vi "Create Server from Template.vi"(8 "error in (no error)":errorcluster, 9 "Generated Server Name":string="Generated Server", 10 "Target Project Path":path, 11 "Application ref in":refnum<vi>) -> (0 "error out":errorcluster, 1 "Already exists ?":bool, 2 "Server class out":refnum<vi>, 3 "Server library out":refnum<vi>)   [LabVIEW 2019, in "gRPC Scripting Tools.lvlib"]
uses:
  gRPC Scripting Tools.lvlib
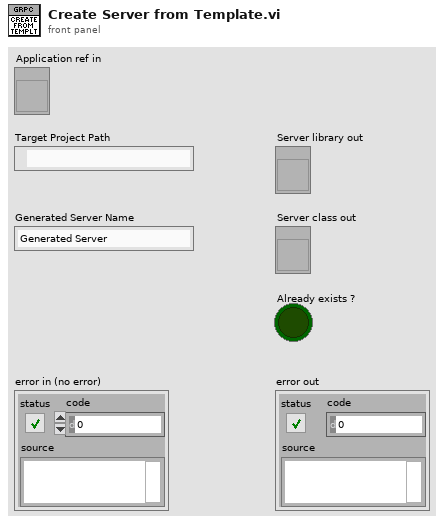
[diagram p1: front panel]
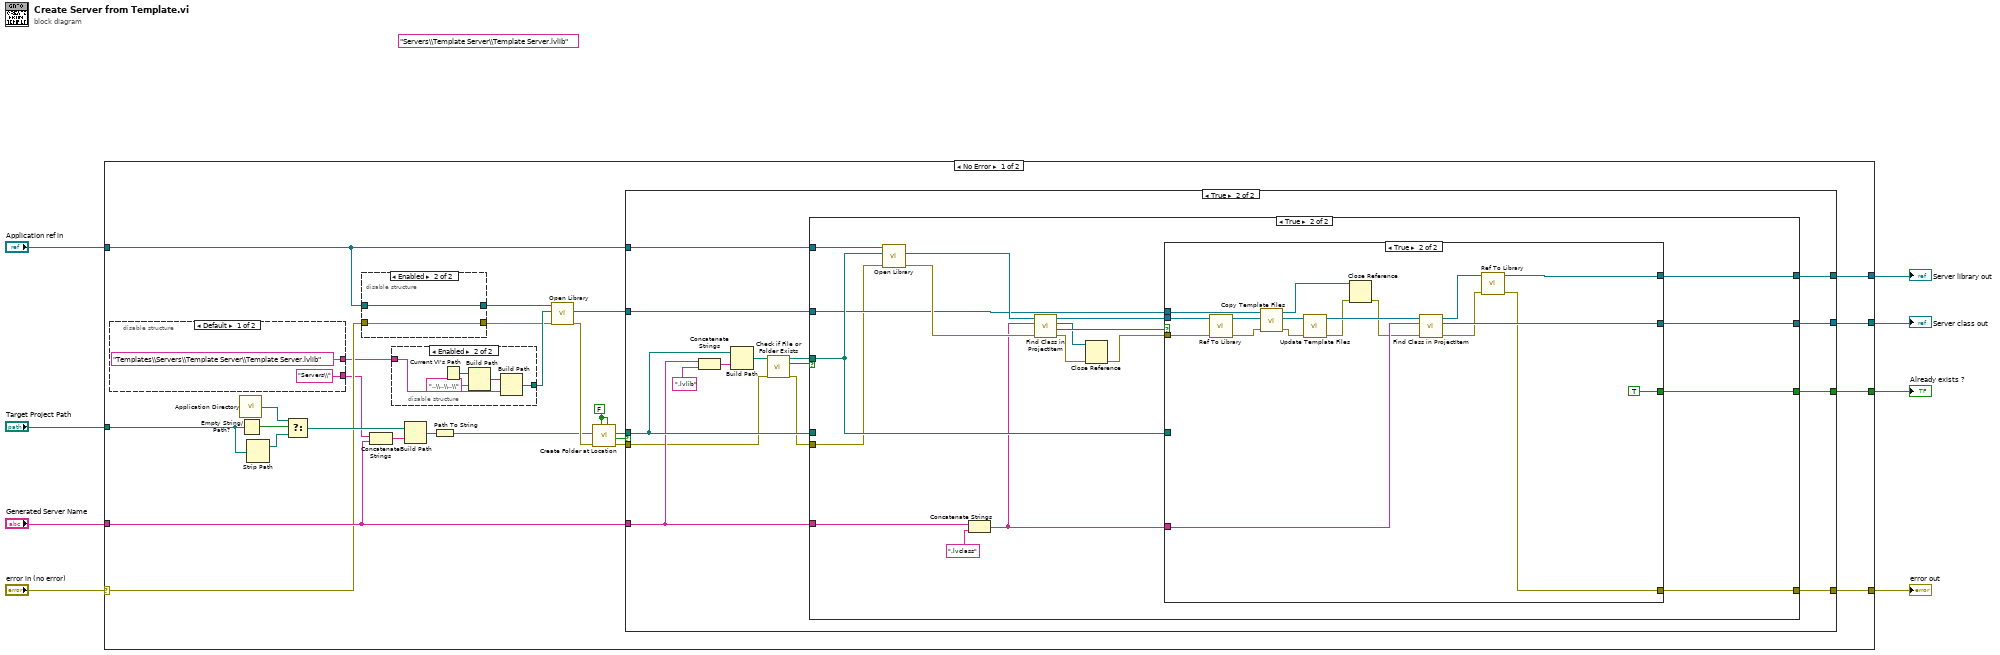
[diagram p0: block diagram]
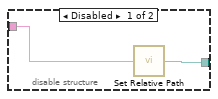
[diagram p2: hidden frame]
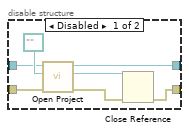
[diagram p3: hidden frame]
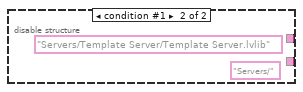
[diagram p4: hidden frame]
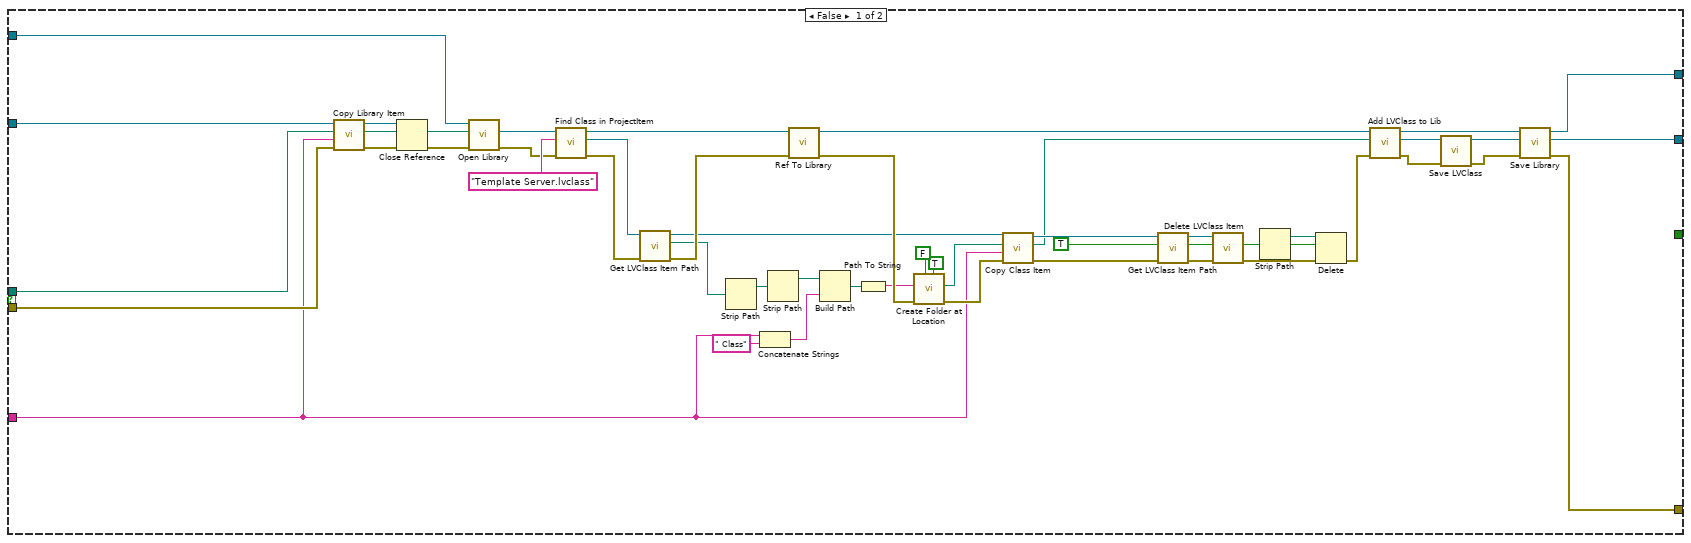
[diagram p5: hidden frame]
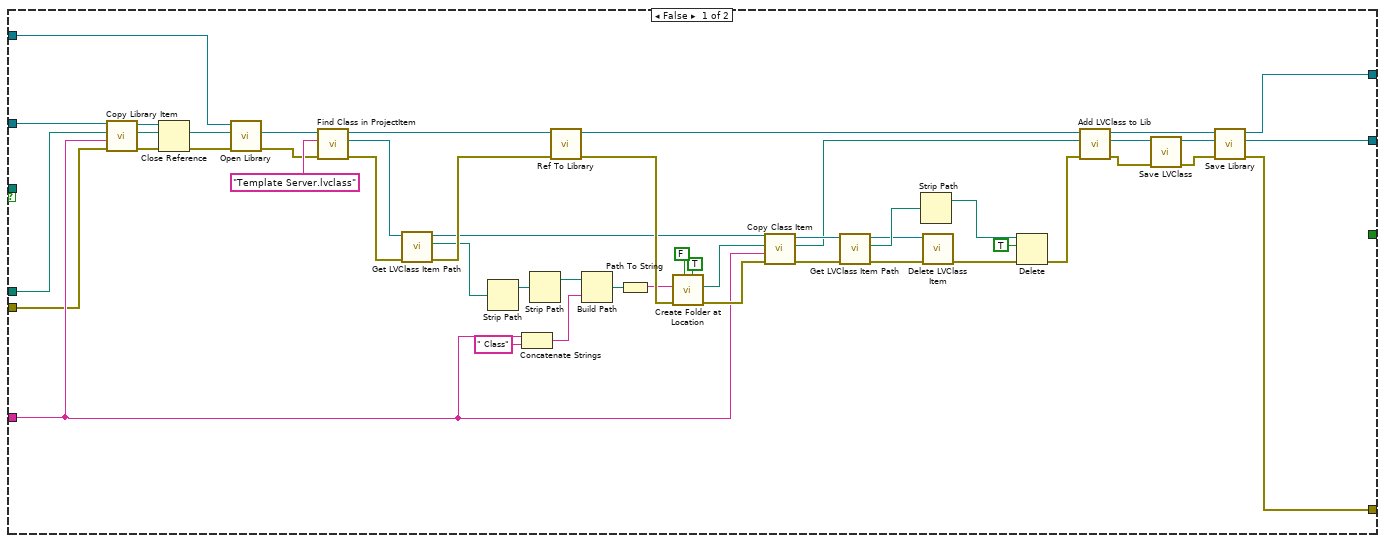
[diagram p6: hidden frame]
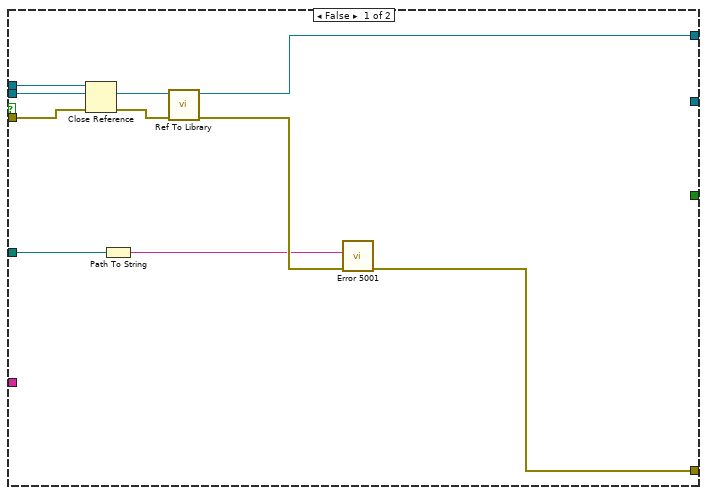
[diagram p7: hidden frame]
diagram:
  (unwired) "Servers\\Template Server\\Template Server.lvlib" ("Application Relative Path")
  n1 = case shown="No Error" "error in (no error)" {
    selector: "error in (no error)" -> [w13 w207]
    tunnel: [w34 w207] -> w8
    tunnel: [w33 _] -> w7
    tunnel: [w32 _] -> w6
    tunnel: "Target Project Path" -> [w16 _]
    tunnel: "Generated Server Name" -> [w15 _]
    tunnel: "Application ref in" -> [w14 _]
    tunnel: [w11 _] -> w1
    frame No Error {
      w25 = FALSE ("Use Relative")
      n2 = disable-structure shown="Default" {
        disable-tunnel: ["Templates\\Servers\\Template Server\\Template Server.lvlib" ("Application Relative Path") _] -> w10
        disable-tunnel: ["Servers\\" ("Path") _] -> w9
        frame condition #0 (active) {
        }
        frame condition #1 {
          (unwired) "Servers/" ("Path")
          (unwired) "Servers/Template Server/Template Server.lvlib" ("Application Relative Path")
        }
      }
      n3 = call <vilib>:"Application Directory.vi"() -> ("Application Directory"=w17:path)
      n4 = Empty String/Path?(string/path=w16) -> (empty?=w20:bool)
      n5 = Strip Path(path=w16) -> (stripped path=w19:path)  [unwired: 1 out]
      n6 = Select(t=w17, s=w20, f=w19) -> (s? t:f=w18:path)
      n7 = disable-structure shown="Enabled" {
        disable-tunnel: [w48 w50] -> w28
        disable-tunnel: [w45 w49] -> w21
        disable-tunnel: w14 -> [w43 w50]
        disable-tunnel: w13 -> [w42 w49]
        frame Disabled {
          n8 = call "Open Project.vi"("error in (no error)"=w42, "Project Path in"=path "", "Application reference"=w43) -> ("error out"=w46:errorcluster, "Project out"=w47:refnum<vi>, "Application out"=w48:refnum<vi>)  [unwired: 6 in]
          n9 = Close Reference(reference=w47, error in (no error)=w46) -> (error out=w45:errorcluster)
        }
        frame Enabled {
        }
      }
      n10 = Concatenate Strings(w9, w15) -> (w24:string)
      n11 = disable-structure shown="Enabled" {
        disable-tunnel: [w36 w39] -> w29
        disable-tunnel: w10 -> [w35 w37]
        frame Disabled {
          n12 = call "Set Relative Path.vi"("Application Relative Path"=w35) -> ("Full Path"=w36:path)
        }
        frame Enabled {
          n13 = Current VI's Path() -> (path=w41:path)
          n14 = Build Path(base path=w41, name or relative path="..\\..\\..\\") -> (appended path=w38:path)
          n15 = Build Path(base path=w38, name or relative path=w37) -> (appended path=w39:path)
        }
      }
      n16 = Build Path(base path=w18, name or relative path=w24) -> (appended path=w23:path)
      n17 = Path To String(path=w23) -> (string=w22:string)
      n18 = call "Open Library.vi"("error in (no error)"=w21, "Full Path"=w29, "Application in"=w28) -> ("error out"=w30:errorcluster, "Library out"=w26:refnum<vi>)  [unwired: 6 in, 1 out]
      n19 = call "Create Folder at Location.vi"("Override existing (F)"=w25, "Use Relative (F)"=w25, "Error In"=w30, "Path"=w22) -> ("Error Out"=w31:errorcluster, "Already Exists ?"=w12:bool, "Full path out"=w27:path)  [unwired: 5 in]
      n20 = case shown="True" w12 {
        tunnel: [w99 w104] -> w34
        tunnel: [w98 w109] -> w33
        tunnel: [w97 w110] -> w32
        tunnel: w31 -> [w61 w101]
        tunnel: w27 -> [w60 w106]
        tunnel: w26 -> [w59 w107]
        tunnel: w15 -> [w54 w105]
        tunnel: w14 -> [w53 w108]
        tunnel: [_ w103] -> w11
        frame False {
          n21 = call "Copy Library Item.vi"("error in (no error)"=w61, "Copy Name"=w54, "Copy location"=w60, "Library in"=w59) -> ("error out"=w82:errorcluster, "New Lib Path"=w58:path, "Library out"=w81:refnum<vi>)  [unwired: 5 in]
          n22 = Close Reference(reference=w81, error in (no error)=w82) -> (error out=w57:errorcluster)
          n23 = call "Open Library.vi"("error in (no error)"=w57, "Full Path"=w58, "Application in"=w53) -> ("error out"=w55:errorcluster, "Library out"=w56:refnum<vi>)  [unwired: 6 in, 1 out]
          n24 = call "Find Class in ProjectItem.vi"("error in (no error)"=w55, "Class Name"="Template Server.lvclass", "ProjectItem in"=w56) -> ("error out"=w64:errorcluster, "LVClass out"=w63:refnum<vi>, "ProjectItem out"=w76:refnum<vi>)  [unwired: 5 in, 1 out]
          n25 = call "Get LVClass Item Path.vi"("error in (no error)"=w64, "LVClassLibrary in"=w63) -> ("error out"=w78:errorcluster, "Path"=w65:path, "LVClassLibrary out"=w66:refnum<vi>)  [unwired: 7 in]
          n26 = Strip Path(path=w65) -> (stripped path=w74:path)  [unwired: 1 out]
          n27 = Concatenate Strings(w54, " Class" ("string")) -> (w69:string)
          n28 = Strip Path(path=w74) -> (stripped path=w75:path)  [unwired: 1 out]
          n29 = call "Ref To Library.vi"("error in (no error)"=w78, "ProjectItem in"=w76) -> ("error out"=w79:errorcluster, "Library out"=w92:refnum<vi>)  [unwired: 8 in]
          n30 = Build Path(base path=w75, name or relative path=w69) -> (appended path=w70:path)
          n31 = Path To String(path=w70) -> (string=w71:string)
          n32 = call "Create Folder at Location.vi"("Override existing (F)"=TRUE, "Use Relative (F)"=FALSE ("Use Relative"), "Error In"=w79, "Path"=w71) -> ("Error Out"=w80:errorcluster, "Full path out"=w73:path)  [unwired: 5 in, 1 out]
          n33 = call "Copy Class Item.vi"("error in (no error)"=w80, "New Name"=w54, "Full path in"=w73, "LVClassLibrary in"=w66) -> ("error out"=w84:errorcluster, "New Class Path out"=w77:path, "LVClassLibrary out"=w83:refnum<vi>)  [unwired: 5 in]
          n34 = call "Get LVClass Item Path.vi"("error in (no error)"=w84, "LVClassLibrary in"=w83) -> ("error out"=w86:errorcluster, "Path"=w87:path, "LVClassLibrary out"=w85:refnum<vi>)  [unwired: 7 in]
          n35 = call "Delete LVClass Item.vi"("error in (no error)"=w86, "LVClassLibrary in"=w85) -> ("error out"=w89:errorcluster)  [unwired: 9 in]
          n36 = Strip Path(path=w87) -> (stripped path=w88:path)  [unwired: 1 out]
          n37 = Delete(path (use dialog)=w88, entire hierarchy (F)=TRUE, error in=w89) -> (error out=w90:errorcluster)  [unwired: 2 in, 2 out]
          n38 = call "Add LVClass to Lib.vi"("error in (no error)"=w90, "LVClass Path in"=w77, "Library in"=w92) -> ("error out"=w95:errorcluster, "LVClassLibrary out"=w94:refnum<vi>, "Library out"=w93:refnum<vi>)  [unwired: 6 in]
          n39 = call "Save LVClass.vi"("error in (no error)"=w95, "LVClassLibrary in"=w94) -> ("error out"=w96:errorcluster, "LVClassLibrary out"=w98:refnum<vi>)  [unwired: 8 in]
          n40 = call "Save Library.vi"("error in (no error)"=w96, "Library in"=w93) -> ("error out"=w99:errorcluster, "Library out"=w97:refnum<vi>)  [unwired: 8 in]
        }
        frame True {
          n41 = Concatenate Strings(w105, ".lvlib" ("string")) -> (w113:string)
          n42 = Build Path(base path=w106, name or relative path=w113) -> (appended path=w112:path)
          n43 = call <vilib>:"Check if File or Folder Exists.vi"("error in (no error)"=w101, "path"=w112) -> ("error out"=w100:errorcluster, "file or folder exists?"=w111:bool, "dup path"=w102:path)  [unwired: 7 in]
          n44 = case shown="True" w111 {
            tunnel: [w122 w173] -> w110
            tunnel: [w121 w162] -> w109
            tunnel: w108 -> [w120 w179]
            tunnel: w107 -> [w119 w168]
            tunnel: w106 -> [w118 _]
            tunnel: w105 -> [w117 w177]
            tunnel: w100 -> [w116 w167]
            tunnel: [w115 w172] -> w104
            tunnel: [_ w170] -> w103
            tunnel: w102 -> [_ w169]
            frame False {
              n45 = call "Copy Library Item.vi"("error in (no error)"=w116, "Copy Name"=w117, "Copy location"=w118, "Library in"=w119) -> ("error out"=w147:errorcluster, "New Lib Path"=w126:path, "Library out"=w146:refnum<vi>)  [unwired: 5 in]
              n46 = Close Reference(reference=w146, error in (no error)=w147) -> (error out=w125:errorcluster)
              n47 = call "Open Library.vi"("error in (no error)"=w125, "Full Path"=w126, "Application in"=w120) -> ("error out"=w123:errorcluster, "Library out"=w124:refnum<vi>)  [unwired: 6 in, 1 out]
              n48 = call "Find Class in ProjectItem.vi"("error in (no error)"=w123, "Class Name"="Template Server.lvclass", "ProjectItem in"=w124) -> ("error out"=w129:errorcluster, "LVClass out"=w128:refnum<vi>, "ProjectItem out"=w141:refnum<vi>)  [unwired: 5 in, 1 out]
              n49 = call "Get LVClass Item Path.vi"("error in (no error)"=w129, "LVClassLibrary in"=w128) -> ("error out"=w143:errorcluster, "Path"=w130:path, "LVClassLibrary out"=w131:refnum<vi>)  [unwired: 7 in]
              n50 = Strip Path(path=w130) -> (stripped path=w139:path)  [unwired: 1 out]
              n51 = Concatenate Strings(w117, " Class" ("string")) -> (w134:string)
              n52 = Strip Path(path=w139) -> (stripped path=w140:path)  [unwired: 1 out]
              n53 = call "Ref To Library.vi"("error in (no error)"=w143, "ProjectItem in"=w141) -> ("error out"=w144:errorcluster, "Library out"=w157:refnum<vi>)  [unwired: 8 in]
              n54 = Build Path(base path=w140, name or relative path=w134) -> (appended path=w135:path)
              n55 = Path To String(path=w135) -> (string=w136:string)
              n56 = call "Create Folder at Location.vi"("Override existing (F)"=TRUE, "Use Relative (F)"=FALSE ("Use Relative"), "Error In"=w144, "Path"=w136) -> ("Error Out"=w145:errorcluster, "Full path out"=w138:path)  [unwired: 5 in, 1 out]
              n57 = call "Copy Class Item.vi"("error in (no error)"=w145, "New Name"=w117, "Full path in"=w138, "LVClassLibrary in"=w131) -> ("error out"=w149:errorcluster, "New Class Path out"=w142:path, "LVClassLibrary out"=w148:refnum<vi>)  [unwired: 5 in]
              n58 = call "Get LVClass Item Path.vi"("error in (no error)"=w149, "LVClassLibrary in"=w148) -> ("error out"=w151:errorcluster, "Path"=w152:path, "LVClassLibrary out"=w150:refnum<vi>)  [unwired: 7 in]
              n59 = Strip Path(path=w152) -> (stripped path=w153:path)  [unwired: 1 out]
              n60 = call "Delete LVClass Item.vi"("error in (no error)"=w151, "LVClassLibrary in"=w150) -> ("error out"=w154:errorcluster)  [unwired: 9 in]
              n61 = Delete(path (use dialog)=w153, entire hierarchy (F)=TRUE, error in=w154) -> (error out=w155:errorcluster)  [unwired: 2 in, 2 out]
              n62 = call "Add LVClass to Lib.vi"("error in (no error)"=w155, "LVClass Path in"=w142, "Library in"=w157) -> ("error out"=w160:errorcluster, "LVClassLibrary out"=w159:refnum<vi>, "Library out"=w158:refnum<vi>)  [unwired: 6 in]
              n63 = call "Save LVClass.vi"("error in (no error)"=w160, "LVClassLibrary in"=w159) -> ("error out"=w161:errorcluster, "LVClassLibrary out"=w121:refnum<vi>)  [unwired: 8 in]
              n64 = call "Save Library.vi"("error in (no error)"=w161, "Library in"=w158) -> ("error out"=w115:errorcluster, "Library out"=w122:refnum<vi>)  [unwired: 8 in]
            }
            frame True {
              n65 = call "Open Library.vi"("error in (no error)"=w167, "Full Path"=w169, "Application in"=w179) -> ("error out"=w175:errorcluster, "Library out"=w178:refnum<vi>)  [unwired: 6 in, 1 out]
              n66 = Concatenate Strings(w177, ".lvclass" ("Class Name")) -> (w163:string)
              n67 = call "Find Class in ProjectItem.vi"("error in (no error)"=w175, "Class Name"=w163, "ProjectItem in"=w178) -> ("error out"=w165:errorcluster, "Found?"=w171:bool, "LVClass out"=w166:refnum<vi>, "ProjectItem out"=w174:refnum<vi>)  [unwired: 5 in]
              n68 = Close Reference(reference=w166, error in (no error)=w165) -> (error out=w164:errorcluster)
              n69 = case shown="True" w171 {
                tunnel: w174 -> [w188 w201]
                tunnel: [w187 w206] -> w173
                tunnel: w164 -> [w182 w203]
                tunnel: [w185 w194] -> w172
                tunnel: w169 -> [w184 _]
                tunnel: [_ TRUE] -> w170
                tunnel: w168 -> [w183 w193]
                tunnel: w163 -> [_ w200]
                tunnel: [_ w199] -> w162
                frame False {
                  n70 = Close Reference(reference=w183, error in (no error)=w182) -> (error out=w181:errorcluster)
                  n71 = Path To String(path=w184) -> (string=w180:string)
                  n72 = call "Ref To Library.vi"("error in (no error)"=w181, "ProjectItem in"=w188) -> ("error out"=w186:errorcluster, "Library out"=w187:refnum<vi>)  [unwired: 8 in]
                  n73 = call "Error 5001.vi"("error in (no error)"=w186, "Server Class Path"=w180) -> ("error out"=w185:errorcluster)  [unwired: 9 in]
                }
                frame True {
                  n74 = call "Ref To Library.vi"("error in (no error)"=w203, "ProjectItem in"=w201) -> ("error out"=w202:errorcluster, "Library out"=w204:refnum<vi>)  [unwired: 8 in]
                  n75 = call "Copy Template Files.vi"("error in (no error)"=w202, "Server Library (Library Item) in"=w204, "Template Library (Library Item) in"=w193) -> ("error out"=w192:errorcluster, "Server Library (Library Item) out"=w191:refnum<vi>, "Template Library (Library Item) out"=w189:refnum<vi>)  [unwired: 6 in]
                  n76 = call "Update Template Files.vi"("error in (no error)"=w192, "Server Library (Library Item) in"=w191) -> ("error out"=w190:errorcluster, "Server Library (Library Item) out"=w198:refnum<vi>)  [unwired: 8 in]
                  n77 = Close Reference(reference=w189, error in (no error)=w190) -> (error out=w196:errorcluster)
                  n78 = call "Find Class in ProjectItem.vi"("error in (no error)"=w196, "Class Name"=w200, "ProjectItem in"=w198) -> ("error out"=w195:errorcluster, "LVClass out"=w199:refnum<vi>, "ProjectItem out"=w197:refnum<vi>)  [unwired: 5 in, 1 out]
                  n79 = call "Ref To Library.vi"("error in (no error)"=w195, "ProjectItem in"=w197) -> ("error out"=w194:errorcluster, "Library out"=w206:refnum<vi>)  [unwired: 8 in]
                }
              }
            }
          }
        }
      }
    }
    frame Error {
    }
  }
  "error out" <- w8
  "Server class out" <- w7
  "Server library out" <- w6
  "Already exists ?" <- w1
